vi "GSM_MEAS_TYPE.vi"(4 "RO":bool, 6 "INST MEAS":T1(ring), 8 "error in":errorcluster {"code" format="%.0x"}, 11 "Session In":refnum<visa-resource-name>="TCPIP0::K-N90X0A-00005.local::hislip0::INSTR") -> (0 "error out":errorcluster {"code" format="%.0x"}, 3 "Session Out":refnum<visa-resource-name>, 5 "meas":string)   [LabVIEW 2018]
panel:
  in  "Timeout":u32=3000
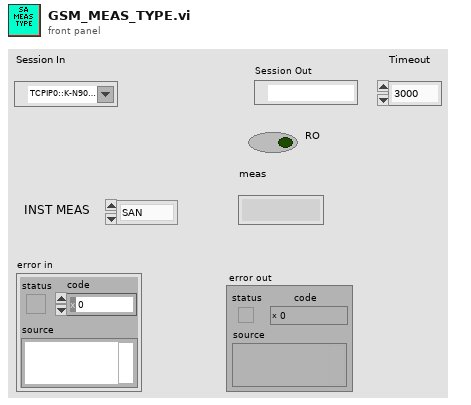
[diagram p1: front panel]
types:
  T1 = enum16{"SAN", "SEM", "CHP", "OBW", "ACP", "PST", "SPUR", "TXP", "TOI", "HARM"}
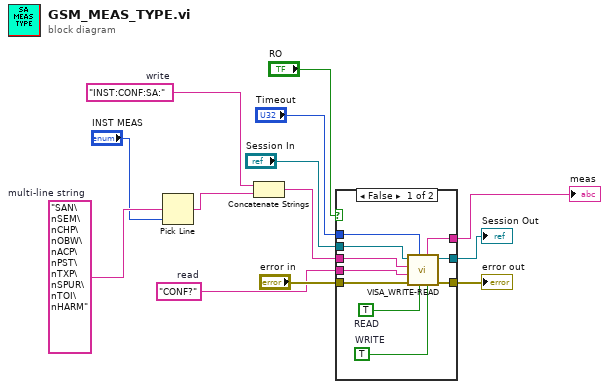
[diagram p0: block diagram]
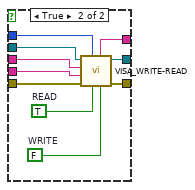
[diagram p2: hidden frame]
diagram:
  w9 = "CONF?"  # read
  w2 = "SAN\nSEM\nCHP\nOBW\nACP\nPST\nTXP\nSPUR\nTOI\nHARM"  # multi-line string
  w11 = "INST:CONF:SA:"  # write
  n1 = Pick Line(multi-line string=w2, line index="INST MEAS") -> (output string=w3:string)  [unwired: 1 in]
  n2 = Concatenate Strings(w11, w3) -> (w10:string)
  n3 = case shown="False" "RO" {
    tunnel: "error in" -> [w23 w33]
    tunnel: [w22 w32] -> w12
    tunnel: w10 -> [w21 w31]
    tunnel: w9 -> [w20 w30]
    tunnel: "Session In" -> [w19 w29]
    tunnel: [w18 w28] -> w7
    tunnel: [w17 w27] -> w4
    tunnel: "Timeout" -> [w16 w26]
    frame False {
      w14 = TRUE  # WRITE
      w15 = TRUE  # READ
      n4 = call "VISA_WRITE-READ.vi"("WRITE"=w14, "READ"=w15, "Timeout"=w16, "error in"=w23, "Rcmd"=w20, "Wcmd"=w21, "Session In"=w19) -> ("error out"=w22:errorcluster, "Session Out"=w18:refnum<visa-resource-name>, "Out"=w17:string)  [unwired: 2 in]
    }
    frame True {
      w24 = FALSE  # WRITE
      w25 = TRUE  # READ
      n5 = call "VISA_WRITE-READ.vi"("WRITE"=w24, "READ"=w25, "Timeout"=w26, "error in"=w33, "Rcmd"=w30, "Wcmd"=w31, "Session In"=w29) -> ("error out"=w32:errorcluster, "Session Out"=w28:refnum<visa-resource-name>, "Out"=w27:string)  [unwired: 2 in]
    }
  }
  "error out" <- w12
  "Session Out" <- w7
  "meas" <- w4
